vi "Memory.Pointer.Internal.Duplicate.vi"(8 "error in (no error)":errorcluster, 10 "new pointer type":refnum<class "Memory.Pointer.Internal.lvclass">, 11 "pointer in":refnum<class "Memory.Pointer.lvclass">) -> (0 "error out":errorcluster, 2 "new pointer":refnum<class "Memory.Pointer.Internal.lvclass">, 3 "pointer out":refnum<class "Memory.Pointer.lvclass">)   [LabVIEW 2016, in "Memory.lvlib" / "Memory.Pointer.Internal.lvclass"]
uses:
  Memory.Pointer.Internal.lvclass
  Pointer/Memory.Pointer.lvclass
  C:/Git/Sourcetree/DSF/Source/Submodules/Memory/Source/Classes/Pointer/Memory.Pointer.lvclass
  Pointer/Memory.Pointer.lvclass/Memory.Pointer.ctl
  Pointer/Memory.Pointer.Copy All.Safe.vi
  Pointer/Memory.Pointer.Copy.Safe.vi
  Pointer/Memory.Pointer.Copy.Unsafe.vi
  Pointer/Memory.Pointer.Parameter Check.Subset.vi
  Pointer/Memory.Pointer.Parameter Check.Null Pointer.vi
  Pointer/Memory.Pointer.Get Address.vi
  Pointer/Memory.Pointer.Errors.vi
  Pointer/Memory.Pointer.Errors.Out of Bounds.vi
  Pointer/Memory.Pointer.Errors.Null Pointer.vi
  Submodules/SEH/Source/VIs/Static Error Handling.Source Buffer.Write.String.vi
  Pointer/Memory.Pointer.Errors.Write Pointer Size.vi
  Pointer/Memory.Pointer.Errors.Create Error.vi
  Submodules/SEH/Source/VIs/Static Error Handling.Source Buffer.Write.Numeric.Scalar.Base10.vi
  Submodules/SEH/Source/VIs/Static Error Handling.Source Buffer.Write.Numeric.Scalar.Base10 (U64).vi
  Submodules/SEH/Source/VIs/Static Error Handling.Error Cluster Constant.vi
  Submodules/SEH/Source/VIs/Static Error Handling.Error Cluster Constant (256B).vi
  Submodules/SEH/Source/VIs/Static Error Handling.Parameters.Status.Set.vi
  Submodules/SEH/Source/VIs/Static Error Handling.Parameters.Code.Set.vi
  Submodules/SEH/Source/VIs/Static Error Handling.Parameters.VI Source.Set.vi
  Constants/Memory.Constants.vi
  Constants/Memory.Constants.Library Name.vi
  Pointer/Memory.Pointer.Errors.Get Info.vi
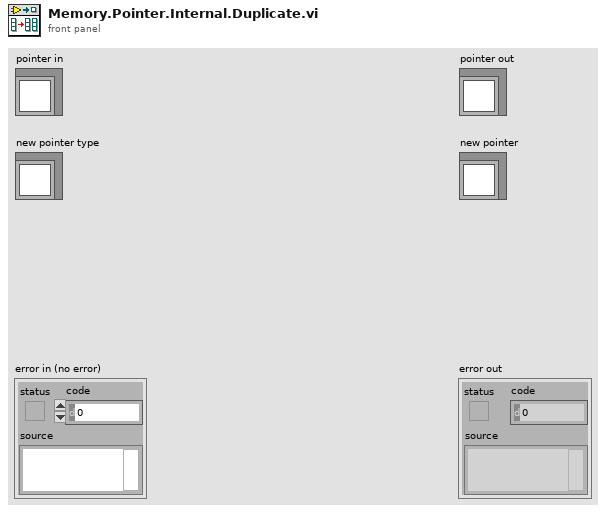
[diagram p1: front panel]
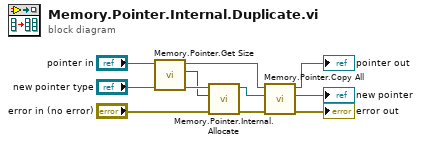
[diagram p0: block diagram]
diagram:
  n1 = call "Memory.Pointer.Get Size.vi"("Pointer in"="pointer in") -> ("size"=w2:u64, "Pointer out"=w8:refnum<class "Memory.Pointer.lvclass">)  [unwired: 9 in]
  n2 = call "Memory.Pointer.Internal.Allocate.vi"("error in (no error)"="error in (no error)", "size"=w2, "pointer in"="new pointer type") -> ("error out"=w10:errorcluster, "pointer out"=w9:refnum<class "Memory.Pointer.Internal.lvclass">)  [unwired: 7 in]
  n3 = call-poly "Memory.Pointer.Copy All.vi"("error in (no error)"=w10, "dst pointer in"=w9, "src pointer in"=w8) -> ("error out"=→"error out":errorcluster, "dst pointer out"=→"new pointer":refnum<class "Memory.Pointer.Internal.lvclass">, "src pointer out"=→"pointer out":refnum<class "Memory.Pointer.lvclass">)  [unwired: 6 in]
